vi "OM3_PreStimCleaning.vi"   [LabVIEW 2015]
uses:
  Intrinsic Rig/software/widefield_imaging_OM2/control_VIs/OM2_control_VIs/global_cleaning_0621.vi
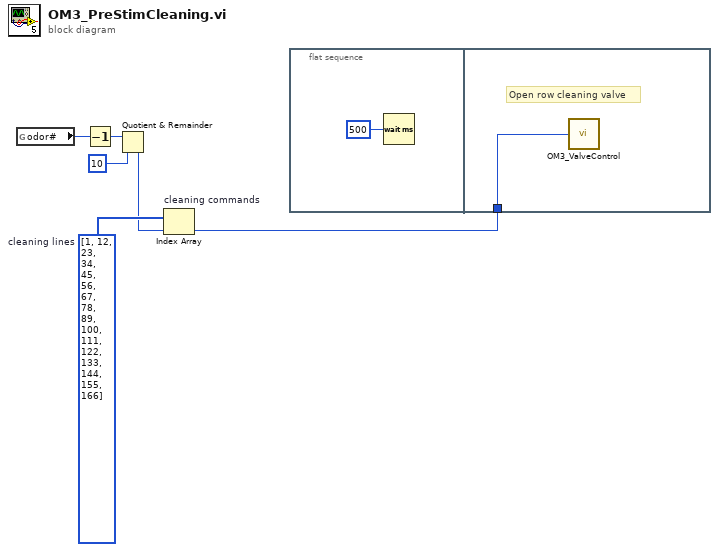
[diagram p0: block diagram]
diagram:
  w6 = i32[] [1, 12, 23, 34, 45, 56, 67, 78, 89, 100, 111, 122, 133, 144, 155, 166]  # cleaning lines
  n1 = global read "global_cleaning_0621.vi" "odor#"() -> (w1:i32)
  n2 = Decrement(x=w1) -> (x-1=w3:i32)
  n3 = Quotient & Remainder(x=w3, y=10) -> (floor(x/y)=w5:i32)  [unwired: 1 out]
  n4 = Index Array "cleaning commands"(array=w6, index=w5) -> (element=w4:i32)
  n5 = flat-sequence {
    tunnel: w4 -> [w8]
    frame #0 {
      n6 = Wait (ms)(milliseconds to wait=u32 500) -> ()  [unwired: 1 out]
    }
    frame #1 {
      # "Open row cleaning valve"
      n7 = call "OM3_ValveControl.vi"("Valve#"=w8) -> ()  [unwired: 1 in]
    }
  }
